vi "Array of Device Info to Channel Data.vi"(1 "Array of Devices":T1[](array[typedef])) -> (0 "Device Channels":i32[](array[numeric]))   [LabVIEW 2014, in "Initialization and IO Node Scripting.lvlib"]
uses:
  Initialization and IO Node Scripting.lvlib
  Controls/Device Information.ctl
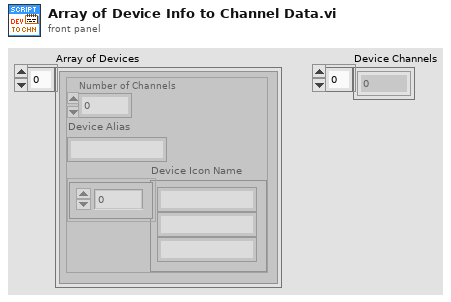
[diagram p1: front panel]
types:
  T1 = typedef "Device Information.ctl" = cluster{"Number of Channels":i32, "Device Alias":string, "Device Icon Name":string[]}
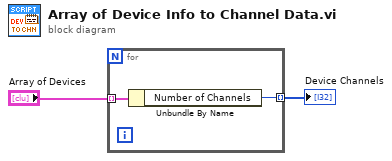
[diagram p0: block diagram]
diagram:
  n1 = for {
    tunnel: "Array of Devices" -> [w4] mode=indexing
    tunnel: [w3] -> w2 mode=indexing
    n2 = Unbundle By Name(w4) -> ("Number of Channels"=w3:i32)
  }
  "Device Channels" <- w2
